vi "Update Alias Name.vi"(7 "Alias Name Ref":refnum<vi>, 8 "error in (no error)":errorcluster, 11 "RESOURCE NAME Ref":refnum<vi>) -> (0 "error out":errorcluster, 3 "Alias Name":string)   [LabVIEW 2025, in "I2C Bus Monitor UI.lvlib"]
uses:
  I2C Bus Monitor UI.lvlib
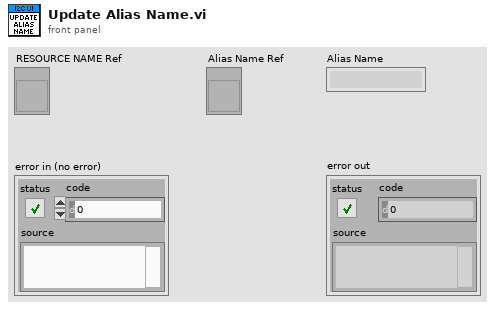
[diagram p1: front panel]
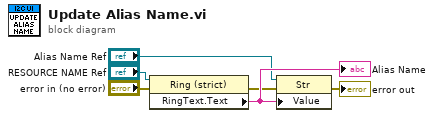
[diagram p0: block diagram]
diagram:
  n1 = property class="Ring (strict)"(reference="RESOURCE NAME Ref", error in="error in (no error)") -> (error out=w4:errorcluster, "RingText.Text"=w6:string)  [unwired: 1 out]
  "Alias Name" <- w6
  n2 = property class="Str"(reference="Alias Name Ref", error in=w4, "Value"=w6) -> (error out=→"error out":errorcluster)  [unwired: 1 out]
